vi "Test Trigger.vi"() -> ()   [LabVIEW 2020]
uses:
  Labview Library/Libraries/HW_LMMR_ASG8100/LMMR ASG/ASG Instructions XControl.xctl
  Labview Library/Libraries/HW_LMMR_ASG8100/LMMR ASG/ASG 8100 Module.lvlib
  Labview Library/Libraries/HW_NI_CTR/NI DAQ Counter/NI DAQ Counter.lvlib
  Labview Library/Libraries/Basic Experiment/Basic Experiment.lvlib
panel:
  out "Data after sum":u32[](array[numeric])
  in  "Loop Number":i32
  out "error out":errorcluster
  in  "\\Delta t":dbl format="%#_5p"
  in  "t_Tr":dbl format="%#_5p"
  in  "test seq":T3(xcontrol)=[{"Flags"=[TRUE, FALSE, FALSE, FALSE, FALSE, FALSE, FALSE, FALSE, FALSE, FALSE, FALSE, FALSE, FALSE, FALSE], "Comments"="", "Time"=2e-06, "Loop Config"={"Loop Code"=enum."Continued", "Number of Loop"=0, "End of Loop"=nan, "Loop Info"=""}}, {"Flags"=[TRUE, FALSE, TRUE, FALSE, FALSE, FALSE, FALSE, FALSE, FALSE, FALSE, FALSE, FALSE, FALSE, FALSE], "Comments"="", "Time"=5e-08, "Loop Config"={"Loop Code"=enum."Continued", "Number of Loop"=0, "End of Loop"=nan, "Loop Info"=""}}, {"Flags"=[TRUE, TRUE, FALSE, FALSE, FALSE, FALSE, FALSE, FALSE, FALSE, FALSE, FALSE, FALSE, FALSE, FALSE], "Comments"="", "Time"=5e-05, "Loop Config"={"Loop Code"=enum."Continued", "Number of Loop"=0, "End of Loop"=nan, "Loop Info"=""}}, {"Flags"=[TRUE, FALSE, TRUE, FALSE, FALSE, FALSE, FALSE, FALSE, FALSE, FALSE, FALSE, FALSE, FALSE, FALSE], "Comments"="", "Time"=5e-08, "Loop Config"={"Loop Code"=enum."Continued", "Number of Loop"=0, "End of Loop"=nan, "Loop Info"=""}}, {"Flags"=[TRUE, FALSE, FALSE, FALSE, FALSE, FALSE, FALSE, FALSE, TRUE, FALSE, FALSE, FALSE, FALSE, FALSE], "Comments"="", "Time"=2e-06, "Loop Config"={"Loop Code"=enum."Continued", "Number of Loop"=0, "End of Loop"=nan, "Loop Info"=""}}, {"Flags"=[TRUE, FALSE, TRUE, FALSE, FALSE, FALSE, FALSE, FALSE, FALSE, FALSE, FALSE, FALSE, FALSE, FALSE], "Comments"="", "Time"=5e-08, "Loop Config"={"Loop Code"=enum."Continued", "Number of Loop"=0, "End of Loop"=nan, "Loop Info"=""}}, {"Flags"=[TRUE, FALSE, FALSE, FALSE, FALSE, FALSE, FALSE, FALSE, FALSE, FALSE, FALSE, FALSE, FALSE, FALSE], "Comments"="", "Time"=5e-05, "Loop Config"={"Loop Code"=enum."Continued", "Number of Loop"=0, "End of Loop"=nan, "Loop Info"=""}}, {"Flags"=[TRUE, FALSE, TRUE, FALSE, FALSE, FALSE, FALSE, FALSE, FALSE, FALSE, FALSE, FALSE, FALSE, FALSE], "Comments"="", "Time"=5e-08, "Loop Config"={"Loop Code"=enum."Continued", "Number of Loop"=0, "End of Loop"=nan, "Loop Info"=""}}, {"Flags"=[TRUE, FALSE, FALSE, FALSE, FALSE, FALSE, FALSE, FALSE, FALSE, FALSE, FALSE, FALSE, FALSE, FALSE], "Comments"="", "Time"=2e-06, "Loop Config"={"Loop Code"=enum."Continued", "Number of Loop"=0, "End of Loop"=nan, "Loop Info"=""}}]
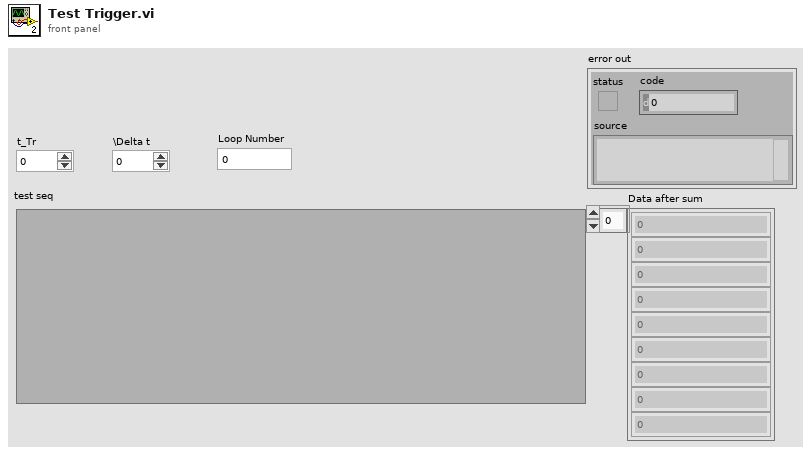
[diagram p1: front panel]
types:
  T1 = typedef "Loop XControl.xctl/Loop Config.ctl" = cluster{"Loop Code":T2, "Number of Loop":i32, "End of Loop":dbl, "Loop Info":string}
  T2 = typedef "Loop XControl.xctl/Loop Code.ctl" = enum16{"Continued", "Loop", "End Loop"}
  T3 = cluster{"Flags":bool[], "Comments":string, "Time":dbl, "Loop Config":T1}[]
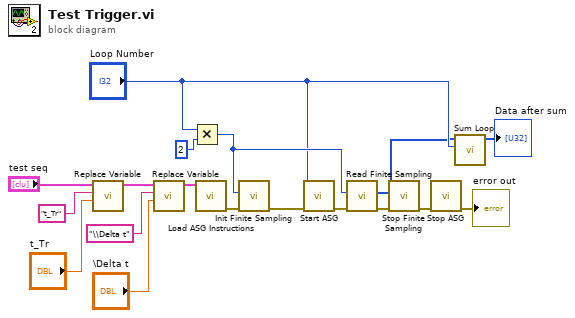
[diagram p0: block diagram]
diagram:
  n1 = call "Replace Variable.vi"("Variable value"="t_Tr", "Variable Name"="t_Tr", "Seq"="test seq") -> ("Result seq"=w14:T3)  [unwired: 8 in]
  n2 = call "Replace Variable.vi"("Variable value"="\\Delta t", "Variable Name"="\\Delta t", "Seq"=w14) -> ("Result seq"=w12:T3)  [unwired: 8 in]
  n3 = Multiply(x="Loop Number", y=2 ("Num of Sample")) -> (x*y=w4:i32)
  n4 = call "Load ASG Instructions.vi"("ASG Instructions"=w12) -> ("error out"=w7:errorcluster)  [unwired: 10 in]
  n5 = call "Init Finite Sampling.vi"("error in"=w7, "Num of Sample"=w4) -> ("error out"=w9:errorcluster)  [unwired: 9 in]
  n6 = call "Start ASG.vi"("error in (no error)"=w9, "Loop Number"="Loop Number") -> ("error out"=w8:errorcluster)  [unwired: 8 in, 1 out]
  n7 = call "Read Finite Sampling.vi"("error in"=w8, "Samples to Read"=w4) -> ("error out"=w11:errorcluster, "Sample Array"=w2:u32[])  [unwired: 7 in, 1 out]
  n8 = call "Stop Finite Sampling.vi"("error in"=w11) -> ("error out"=w10:errorcluster)  [unwired: 10 in]
  n9 = call "Stop ASG.vi"("error in (no error)"=w10) -> ("error out"=→"error out":errorcluster)  [unwired: 9 in, 1 out]
  n10 = call "Sum Loop.vi"("Loop per Update"="Loop Number", "Raw Data Array"=w2) -> ("Data after sum"=→"Data after sum":u32[])  [unwired: 9 in]
